vi "Test Copy Image ARGB Mask ARGB.vi"(8 "error in (no error)":errorcluster, 11 "Test Case In":refnum<class "Image.lvclass">) -> (0 "error out":errorcluster, 3 "Test Case Out":refnum<class "Image.lvclass">)   [LabVIEW 2020, in "g_ar_toolkit.test.lvlib" / "Image.lvclass"]
uses:
  Image.lvclass
  C:/Program Files (x86)/National Instruments/LabVIEW 2020/vi.lib/Astemes/LUnit/Test Case.lvclass
  g_ar_toolkit.common/Image Size (Integer).ctl
  <vilib>/Astemes/LUnit/Test Case.lvclass/Test Case.ctl
  g_ar_toolkit.image/New Image (ARGB).vi
  g_ar_toolkit.image/Copy Array to Image (ARGB).vi
  g_ar_toolkit.image/Copy Image (ARGB with ARGB Mask).vi
  4993e8ee-a06a-463a-9684-69129f64d5ce.vi
  g_ar_toolkit.image/New Image (ARGB).vi/3321fa97-f432-4e1e-8db9-a0df79aed21b.vi
  g_ar_toolkit.image/ARGB Colour to U32 Pixel Value.vi
  g_ar_toolkit.image/Copy Image (ARGB with ARGB Mask).vi/3b1fb24f-4521-4d3d-a8b9-ed3d08148c99.vi
  <vilib>/Astemes/LUnit/Append Pass Result.vi
  <vilib>/Astemes/LUnit/Append Fail Result.vi
  <vilib>/Astemes/LUnit/Describe Comparison.vi
  4993e8ee-a06a-463a-9684-69129f64d5ce.vi/9c5d11cd-9439-4240-a1ee-d9baace9c924.vi
  <vilib>/Astemes/LUnit/Run In UI.vi
  <vilib>/Utility/error.llb/Clear Errors.vi
  g_ar_toolkit.common/Module Path.vi
  <vilib>/Utility/error.llb/Error Cluster From Error Code.vi
  <vilib>/picture/pixmap.llb/Flatten Pixmap.vi
  <vilib>/Astemes/LUnit/Describe Variant.vi
  Image.lvclass/Image.ctl
  g_ar_toolkit.image/g_ar_toolkit.image.lvlib
  g_ar_toolkit.common/g_ar_toolkit.common.lvlib
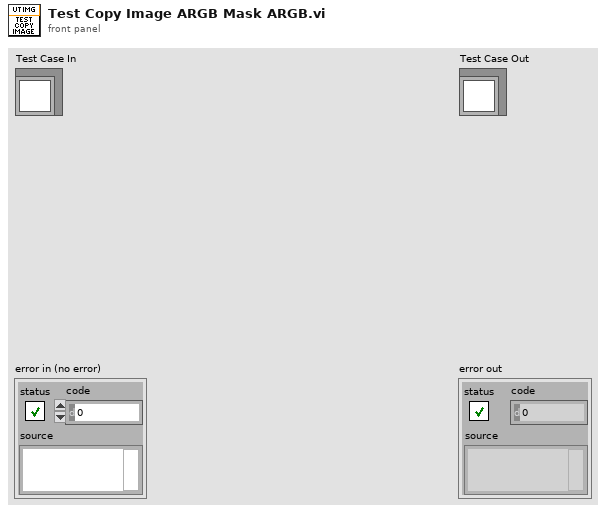
[diagram p1: front panel]
types:
  T1 = typedef "g_ar_toolkit.common.lvlib/Image Size (Integer).ctl" = cluster{"Width":u16, "Height":u16}
  T2 = typedef "g_ar_toolkit.image.lvlib/ARGB Image.ctl" = refnum<data-value>
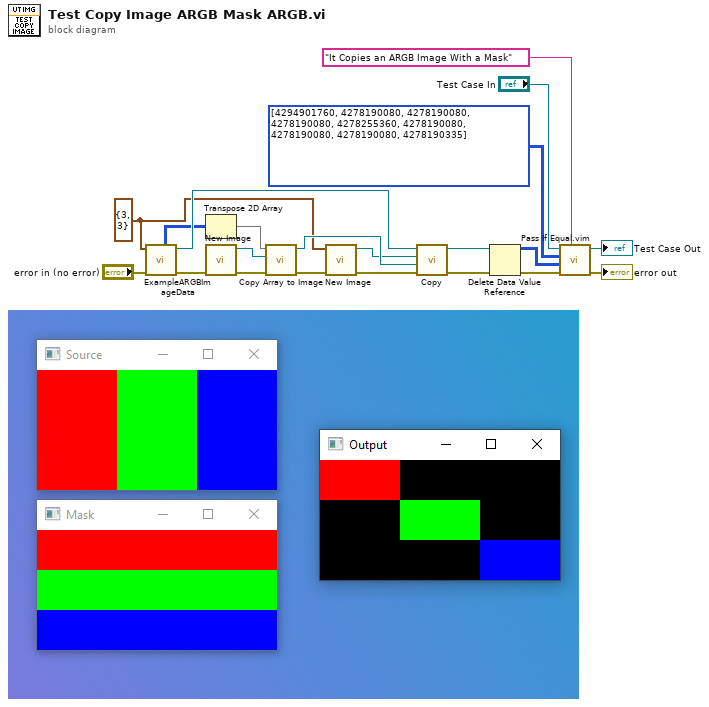
[diagram p0: block diagram]
diagram:
  w3 = T1 {"Width"=3, "Height"=3} ("Preallocated Image Size (Default - 0,0)")
  n1 = call "ExampleARGBImageData.vi"("error in (no error)"="error in (no error)", "Image Size"=w3) -> ("error out"=w16:errorcluster, "Data Value Reference out"=w14:T2, "ARGB Array Data"=w12:u32[][])  [unwired: 6 in, 1 out]
  n2 = Transpose 2D Array(2D array=w12) -> (transposed array=w9:u32[][])
  n3 = call-poly "New Image.vi"("error in (no error)"=w16) -> ("error out"=w11:errorcluster, "New ARGB Image"=w8:T2)  [unwired: 9 in]
  n4 = call-poly "Copy Array to Image.vi"("error in (no error)"=w11, "ARGB Image Destination"=w8, "U32 ARBG Data"=w9) -> ("error out"=w10:errorcluster, "ARGB Image Destination (Duplicate)"=w7:T2)  [unwired: 7 in]
  n5 = call-poly "New Image.vi"("error in (no error)"=w10, "Preallocated Image Size (Default: 0,0)"=w3) -> ("error out"=w5:errorcluster, "New ARGB Image"=w6:T2)  [unwired: 8 in]
  n6 = call-poly "Copy.vi"("error in (no error)"=w5, "ARGB Image Mask"=w7, "ARGB Image Destination"=w6, "ARGB Image Source"=w14) -> ("error out"=w4:errorcluster, "ARGB Image Destination (duplicate)"=w13:T2)  [unwired: 6 in]
  n7 = Delete Data Value Reference(data value reference=w13, error in=w4) -> (data value=w2:u32[][], error out=w15:errorcluster)
  n8 = call "Pass If Equal.vim"("Description"="It Copies an ARGB Image With a Mask", "error in (no error)"=w15, "Actual"=w2, "Expected"=u32[][] [[4294901760, 4278190080, 4278190080], [4278190080, 4278255360, 4278190080], [4278190080, 4278190080, 4278190335]] ("data value"), "LUnit Test Case In"="Test Case In") -> ("error out"=→"error out":errorcluster, "LUnit Test Case Out"=→"Test Case Out":refnum<class "Image.lvclass">)  [unwired: 5 in]
